vi "Preview_Build.vi"(8 "error in (no error)":errorcluster, 11 "Build in":refnum<class "AB_DLL.lvclass">) -> (0 "error out":errorcluster, 1 "GeneratedFiles":path[](array[path]), 3 "Build out":refnum<class "AB_DLL.lvclass">, 4 "GeneratedFileGUIDs":string[](array[string]), 5 "OutputDirectory":path)   [LabVIEW 2020, in "AB_DLL.lvclass"]
uses:
  <vilib>/AppBuilder/AB_Classes/DLL/AB_DLL.lvclass
  e:/builds/penguin/labview/branches/2020/dev/dist/vi.lib/AppBuilder/AB_Classes/Build/AB_Build.lvclass
  e:/builds/penguin/labview/branches/2020/dev/dist/vi.lib/AppBuilder/AB_Classes/TargetFile/AB_Targetfile.lvclass
  <vilib>/AppBuilder/AB_Classes/DLL/AB_DLL.lvclass/AB_DLL.ctl
  <vilib>/AppBuilder/AB_Classes/Application/AB_Application.lvclass
  <vilib>/AppBuilder/AB_Classes/TargetFile/AB_Targetfile.lvclass
  <vilib>/AppBuilder/AB_Classes/Build/AB_Build.lvclass
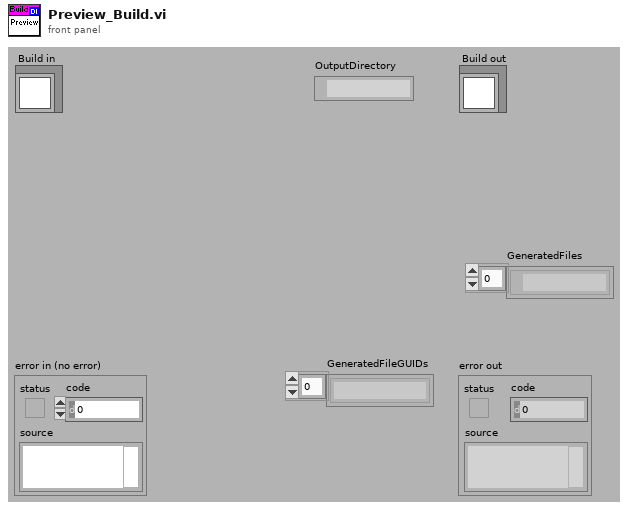
[diagram p1: front panel]
types:
  T1 = enum32{"invalid OS target", "Mac OS", "Windows 3.1", "Windows 95/NT", "Solaris 1", "Solaris 2", "HP-UX", "PowerMAX", "Linux", "Irix", "Rhapsody", "BeOS", "AIX", "OSF1", "VxWorks", "PharLap", "Carbon", "RTX", "Windows x64", "Linux x64", "Mac OS X x64"}
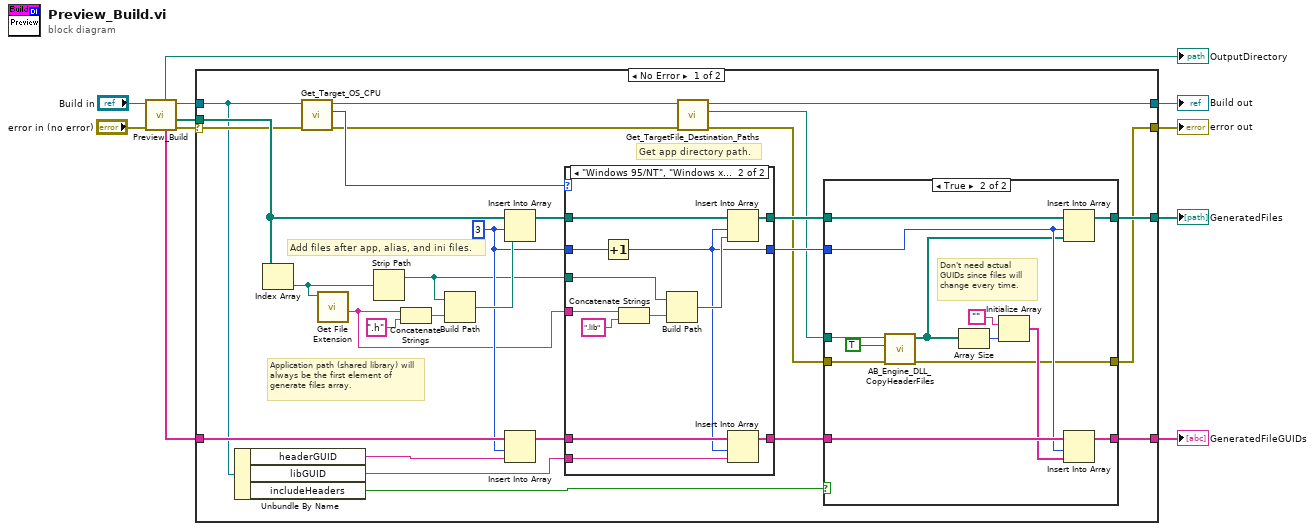
[diagram p0: block diagram]
diagram:
  n1 = call-parent "Preview_Build.vi"("error in (no error)"="error in (no error)", "Build in"="Build in") -> ("error out"=w1:errorcluster, "GeneratedFiles"=w7:path[], "Build out"=w6:refnum<class "AB_DLL.lvclass">, "GeneratedFileGUIDs"=w8:string[], "OutputDirectory"=→"OutputDirectory":path)  [unwired: 5 in]
  n2 = case shown="No Error" w1 {
    selector: w1 -> [w15 w73]
    tunnel: w8 -> [w35 w71]
    tunnel: w7 -> [w33 w72]
    tunnel: w6 -> [w13 w74]
    tunnel: [w18 w74] -> w5
    tunnel: [w23 w72] -> w4
    tunnel: [w22 w71] -> w3
    tunnel: [w21 w73] -> w2
    frame No Error {
      w31 = 3 ("index")
      # "Add files after app, alias, and ini files."
      # "Get app directory path."
      # "Application path (shared library) will always be the first element of generate files array."
      n3 = Unbundle By Name(w13) -> ("headerGUID"=w34:string, "libGUID"=w28:string, "includeHeaders"=w26:bool)
      n4 = Index Array(array=w33) -> (element=w36:path)  [unwired: 1 in]
      n5 = call <vilib>:"Get_Target_OS_CPU.vi"("error in (no error)"=w15, "AB_Build in"=w13) -> ("error out"=w14:errorcluster, "Target Operating System"=w16:T1, "AB_Build out"=w12:refnum<class "AB_DLL.lvclass">)  [unwired: 6 in, 1 out]
      n6 = call <vilib>:"Get File Extension.vi"("file"=w36) -> ("filename without extension"=w27:string)  [unwired: 6 in, 4 out]
      n7 = Strip Path(path=w36) -> (stripped path=w29:path)  [unwired: 1 out]
      n8 = Concatenate Strings(w27, ".h" ("string")) -> (w38:string)
      n9 = Build Path(base path=w29, name or relative path=w38) -> (appended path=w37:path)
      n10 = Insert Into Array(array=w33, index=w31, new element=w37) -> (w32:path[])
      n11 = Insert Into Array(array=w35, index=w31, new element=w34) -> (w30:string[])
      n12 = case shown="\"Windows 95/NT\", \"Windows x64\"" w16 {
        tunnel: w32 -> [w58 w67]
        tunnel: w31 -> [w56 w63]
        tunnel: [w58 w66] -> w25
        tunnel: w30 -> [w57 w65]
        tunnel: [w57 w64] -> w24
        tunnel: w27 -> [_ w69]
        tunnel: w29 -> [_ w68]
        tunnel: w28 -> [_ w61]
        tunnel: [w56 w59] -> w20
        frame Default {
        }
        frame "Windows 95/NT", "Windows x64" {
          n13 = Increment(x=w63) -> (x+1=w59:i32)
          n14 = Concatenate Strings(w69, ".lib" ("string")) -> (w70:string)
          n15 = Build Path(base path=w68, name or relative path=w70) -> (appended path=w62:path)
          n16 = Insert Into Array(array=w67, index=w59, new element=w62) -> (w66:path[])
          n17 = Insert Into Array(array=w65, index=w59, new element=w61) -> (w64:string[])
        }
      }
      n18 = call <vilib>:"Get_TargetFile_Destination_Paths.vi"("error in (no error)"=w14, "AB_Targetfile in"=w12) -> ("error out"=w17:errorcluster, "destination path"=w19:path, "AB_Targetfile out"=w18:refnum<class "AB_DLL.lvclass">)  [unwired: 5 in, 2 out]
      n19 = case shown="True" w26 {
        tunnel: w19 -> [_ w44]
        tunnel: w25 -> [w42 w55]
        tunnel: w24 -> [w41 w53]
        tunnel: [w42 w54] -> w23
        tunnel: [w41 w52] -> w22
        tunnel: w17 -> [w40 w47]
        tunnel: [w40 w46] -> w21
        tunnel: w20 -> [_ w51]
        frame False {
        }
        frame True {
          # "Don't need actual GUIDs since files will change every time."
          n20 = call <vilib>:"AB_Engine_DLL_CopyHeaderFiles.vi"("error in (no error)"=w47, "Preview?"=TRUE ("Preview"), "Path"=w44) -> ("error out"=w46:errorcluster, "GeneratedFiles"=w45:path[])  [unwired: 7 in]
          n21 = Array Size(array=w45) -> (size(s)=w50:i32)
          n22 = Initialize Array("", w50) -> (w48:string[])
          n23 = Insert Into Array(array=w55, index=w51, new element=w45) -> (w54:path[])
          n24 = Insert Into Array(array=w53, index=w51, new element=w48) -> (w52:string[])
        }
      }
    }
    frame Error {
    }
  }
  "error out" <- w2
  "GeneratedFiles" <- w4
  "Build out" <- w5
  "GeneratedFileGUIDs" <- w3
